vi "2D_Array_DualSort.vi"(0 "RawArray":string[][](array[string]), 7 "PrimarySortColumn":i32, 11 "SubSortColumn":i32) -> (4 "SortedArray":string[][](array[string]))   [LabVIEW 2013]
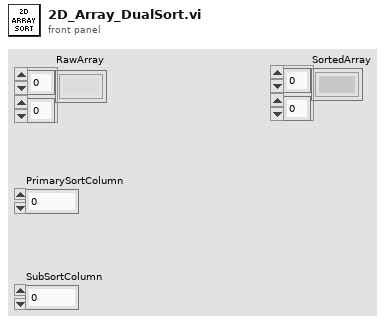
[diagram p1: front panel]
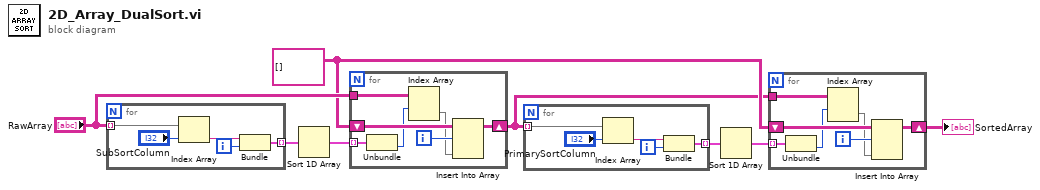
[diagram p0: block diagram]
diagram:
  w3 = string[][] []
  n1 = for {
    tunnel: "RawArray" -> [w12] mode=indexing
    tunnel: [w13] -> w8 mode=indexing
    i -> [w9]
    n2 = Index Array(array=w12, index="SubSortColumn") -> (element=w11:string)
    n3 = Bundle("String"=w11, w9) -> (w13:cluster{"String":string, i32})  [unwired: 1 in]
  }
  n4 = Sort 1D Array(array=w8) -> (sorted array=w6:cluster{"String":string, i32}[])
  n5 = for {
    tunnel: "RawArray" -> [w17]
    shift-right: [w19] -> w2
    shift-left: w3 -> [w20]
    tunnel: w6 -> [w16] mode=indexing
    i -> [w18]
    n6 = Unbundle(w16) -> (w15:i32)  [unwired: 1 out]
    n7 = Index Array(array=w17, index (row)=w15) -> (element=w14:string[])  [unwired: 1 in]
    n8 = Insert Into Array(array=w20, index (row)=w18, new element=w14) -> (w19:string[][])  [unwired: 1 in]
  }
  n9 = for {
    tunnel: w2 -> [w24] mode=indexing
    tunnel: [w25] -> w5 mode=indexing
    i -> [w22]
    n10 = Index Array(array=w24, index="PrimarySortColumn") -> (element=w23:string)
    n11 = Bundle(w23, w22) -> (w25:cluster{string, i32})  [unwired: 1 in]
  }
  n12 = Sort 1D Array(array=w5) -> (sorted array=w4:cluster{string, i32}[])
  n13 = for {
    tunnel: w2 -> [w29]
    shift-right: [w31] -> w1
    shift-left: w3 -> [w32]
    tunnel: w4 -> [w28] mode=indexing
    i -> [w30]
    n14 = Unbundle(w28) -> (w27:i32)  [unwired: 1 out]
    n15 = Index Array(array=w29, index (row)=w27) -> (element=w26:string[])  [unwired: 1 in]
    n16 = Insert Into Array(array=w32, index (row)=w30, new element=w26) -> (w31:string[][])  [unwired: 1 in]
  }
  "SortedArray" <- w1
